vi "setupVersion_June30.vi"() -> (2 "Keithley 2100 out":bool, 3 "Keithley 6431":bool, 4 "J-KEM2":bool, 6 "Keithley 2421":bool, 8 "SRS QCM 2":bool, 10 "OK":bool, 12 "Arduino2":bool, 14 "Pressure control 2":bool, 15 "error IO":errorcluster)   [LabVIEW 2014]
panel:
  in  "ok":bool
  in  "cancel":bool
  in  "Instruments connected":T1
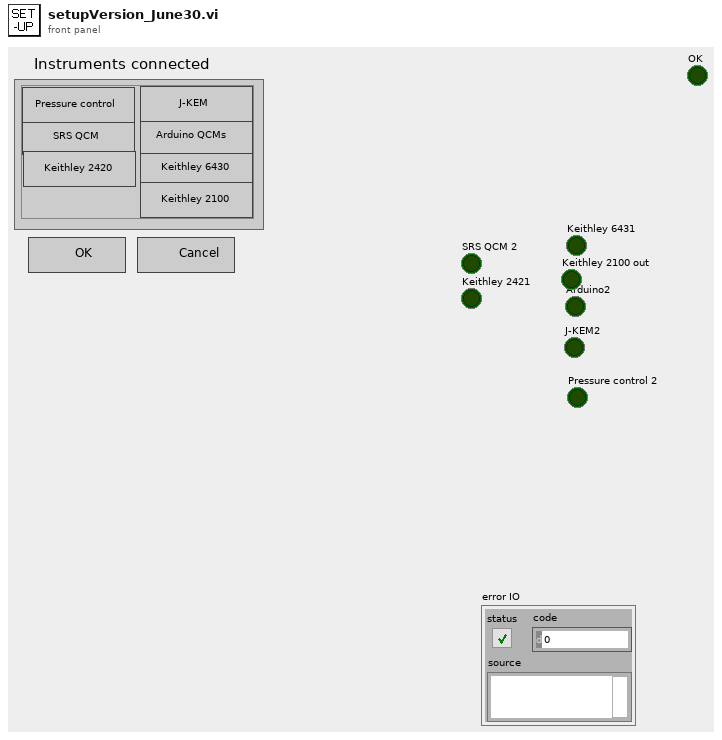
[diagram p1: front panel]
types:
  T1 = cluster{"SRS QCM":bool, "Keithley 2420":bool, "Keithley 6430":bool, "Keithley 2100":bool, "Arduino":bool, "J-KEM":bool, "Pressure control":bool}
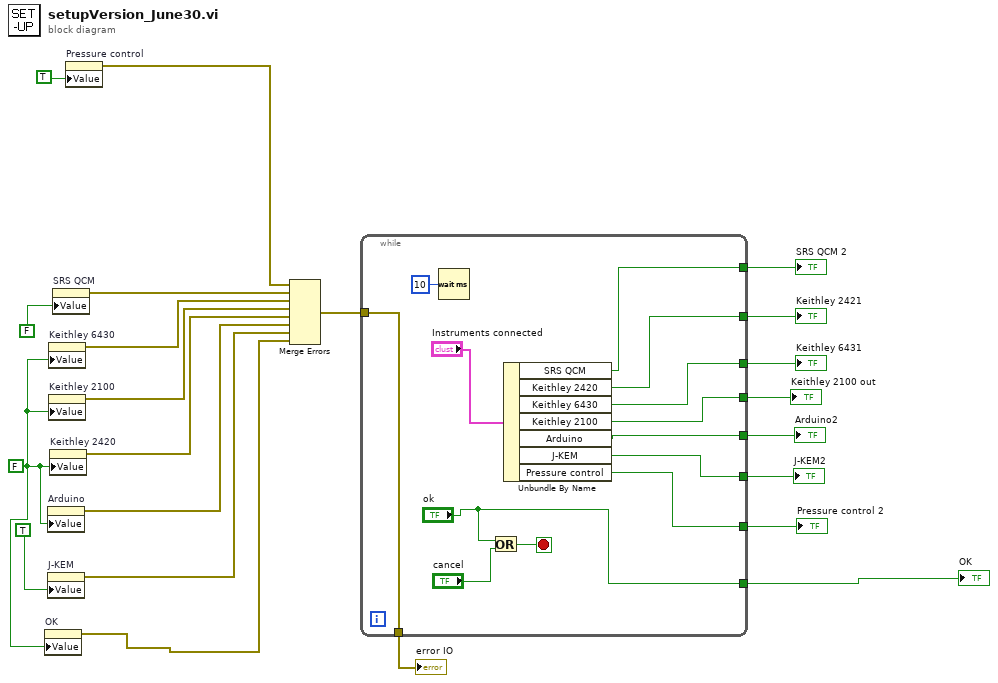
[diagram p0: block diagram]
diagram:
  w2 = FALSE ("Auto Stop")
  n1 = property on="OK" class="Bool (strict)"("Value"=w2) -> (error out=w1:errorcluster)  [unwired: 2 in, 1 out]
  n2 = property on="Arduino" class="Bool (strict)"("Value"=w2) -> (error out=w13:errorcluster)  [unwired: 2 in, 1 out]
  n3 = property on="J-KEM" class="Bool (strict)"("Value"=TRUE ("Auto Stop")) -> (error out=w11:errorcluster)  [unwired: 2 in, 1 out]
  n4 = property on="Keithley 6430" class="Bool (strict)"("Value"=w2) -> (error out=w15:errorcluster)  [unwired: 2 in, 1 out]
  n5 = property on="Keithley 2100" class="Bool (strict)"("Value"=w2) -> (error out=w4:errorcluster)  [unwired: 2 in, 1 out]
  n6 = property on="Keithley 2420" class="Bool (strict)"("Value"=w2) -> (error out=w17:errorcluster)  [unwired: 2 in, 1 out]
  n7 = property on="SRS QCM" class="Bool (strict)"("Value"=FALSE ("Auto Stop")) -> (error out=w14:errorcluster)  [unwired: 2 in, 1 out]
  n8 = property on="Pressure control" class="Bool (strict)"("Value"=TRUE ("Auto Stop")) -> (error out=w6:errorcluster)  [unwired: 2 in, 1 out]
  n9 = Merge Errors(w6, w14, w15, w4, w17, w13, w11, w1) -> (w22:errorcluster)
  n10 = while {
    tunnel: w22 -> [w34]
    tunnel: [w32] -> w21
    tunnel: [w31] -> w20
    tunnel: [w30] -> w19
    tunnel: [w28] -> w18
    tunnel: [w27] -> w12
    tunnel: [w26] -> w9
    tunnel: [w34] -> w7
    tunnel: [w29] -> w5
    tunnel: ["ok"] -> w3
    stop <- w24 stop-if-true
    n11 = Wait (ms)(milliseconds to wait=u32 10) -> ()  [unwired: 1 out]
    n12 = Or(x="ok", y="cancel") -> (x .or. y?=w24:bool)
    n13 = Unbundle By Name("Instruments connected") -> ("SRS QCM"=w32:bool, "Keithley 2420"=w31:bool, "Keithley 6430"=w30:bool, "Keithley 2100"=w29:bool, "Arduino"=w28:bool, "J-KEM"=w27:bool, "Pressure control"=w26:bool)
  }
  "SRS QCM 2" <- w21
  "Keithley 2421" <- w20
  "Keithley 6431" <- w19
  "Arduino2" <- w18
  "J-KEM2" <- w12
  "Pressure control 2" <- w9
  "error IO" <- w7
  "Keithley 2100 out" <- w5
  "OK" <- w3
